vi "decoder.vi"(6 "Mask":dbl[][](array[numeric]), 9 "M":i8, 10 "pulse duration[sample]":i32, 11 "input signal":dbl[](array[numeric])) -> (2 "Array out":i32[](array[numeric]), 3 "residual samples":dbl[](array[numeric]))   [LabVIEW 2017]
uses:
  <vilib>/Analysis/baseanly.llb/Real Dot Product.vi
  <vilib>/Analysis/NI_AALBase.lvlib
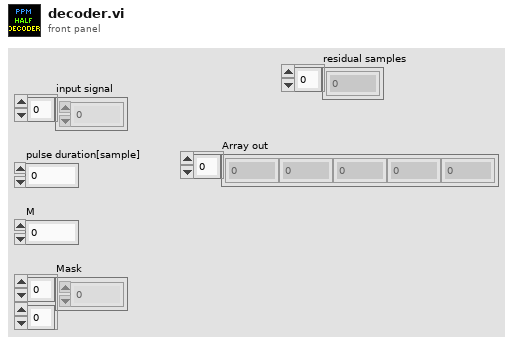
[diagram p1: front panel]
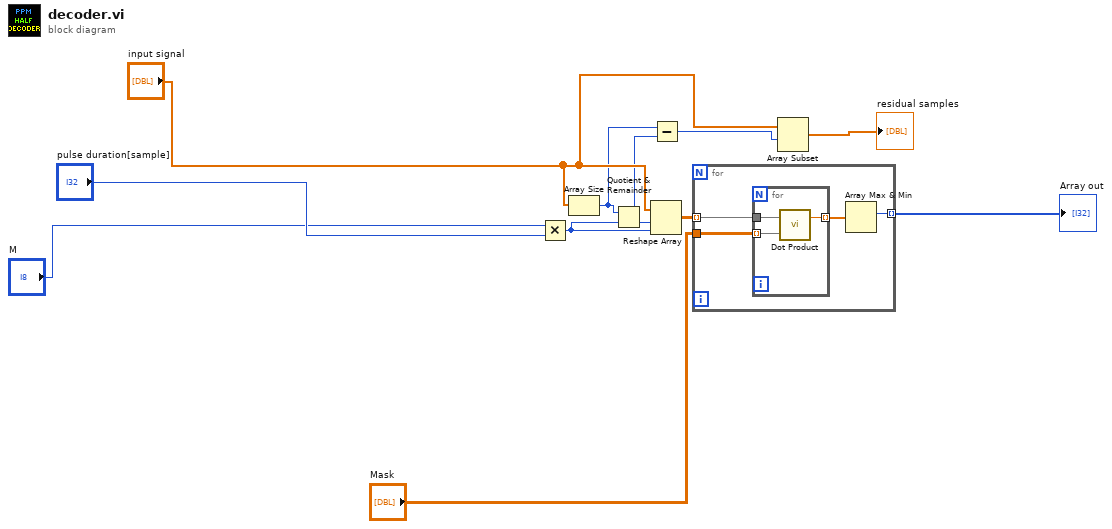
[diagram p0: block diagram]
diagram:
  n1 = Multiply(x="M", y="pulse duration[sample]") -> (x*y=w10:i32)
  n2 = Array Size(array="input signal") -> (size(s)=w3:i32)
  n3 = Quotient & Remainder(x=w3, y=w10) -> (x-y*floor(x/y)=w2:i32, floor(x/y)=w11:i32)
  n4 = Reshape Array("input signal", w11, w10) -> (w6:dbl[][])
  n5 = Subtract(x=w3, y=w2) -> (x-y=w1:i32)
  n6 = for {
    tunnel: w6 -> [w16] mode=indexing
    tunnel: "Mask" -> [w15]
    tunnel: [w13] -> w12 mode=indexing
    n7 = for {
      tunnel: w16 -> [w19]
      tunnel: w15 -> [w18] mode=indexing
      tunnel: [w17] -> w14 mode=indexing
      n8 = call-poly <vilib>:"Dot Product.vi"("Y Vector"=w18, "X Vector"=w19) -> ("X * Y"=w17:dbl)  [unwired: 1 out]
    }
    n9 = Array Max & Min(array=w14) -> (max index (indices)=w13:i32)  [unwired: 3 out]
  }
  "Array out" <- w12
  n10 = Array Subset(array="input signal", index=w1) -> (→"residual samples":dbl[])  [unwired: 1 in]
